vi "SetSRCreationDateStart(SubVI).vi"(10 "Date":timestamp, 11 "HTTP string":string) -> (3 "result string":string)   [LabVIEW 2018, in "Controller.lvlib"]
uses:
  Controller.lvlib
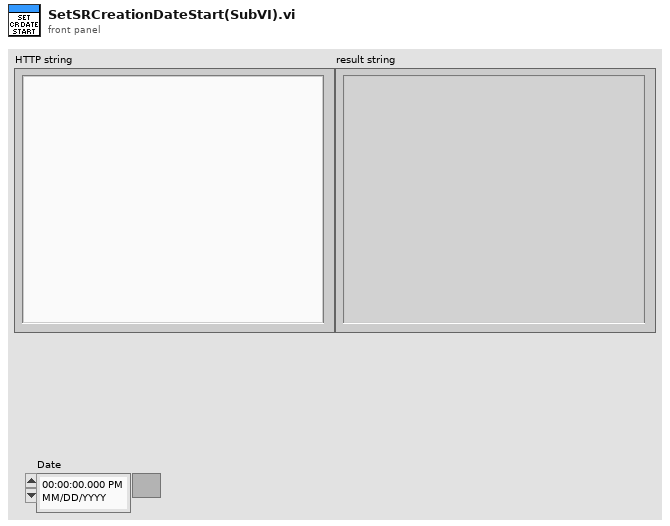
[diagram p1: front panel]
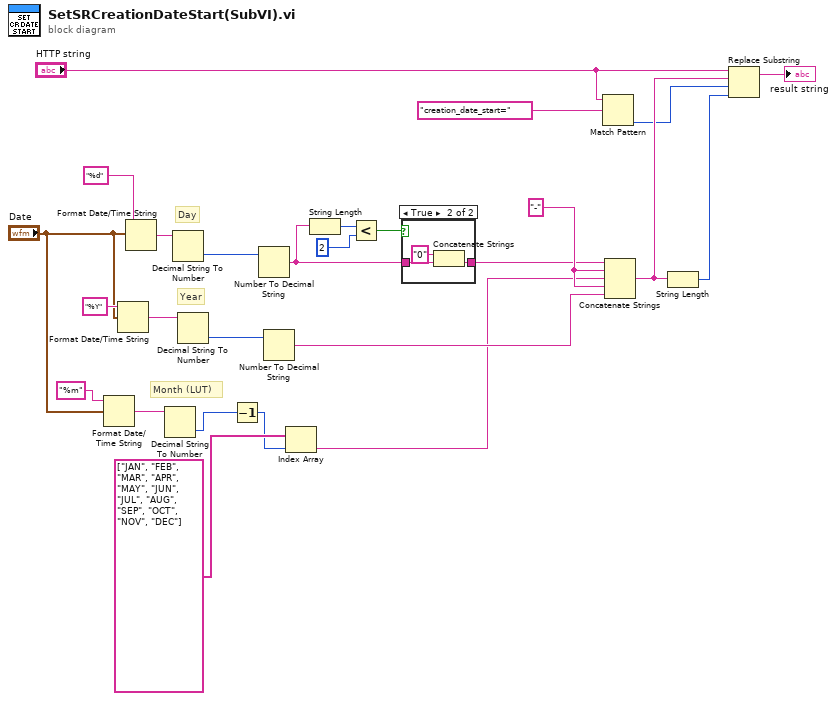
[diagram p0: block diagram]
diagram:
  w20 = "-" ("string")
  # "Month (LUT)"
  # "Year"
  # "Day"
  n1 = Format Date/Time String(time format string (%c)="%m", seconds (now)="Date") -> (date/time string=w6:string)  [unwired: 1 in]
  n2 = Format Date/Time String(time format string (%c)="%Y", seconds (now)="Date") -> (date/time string=w23:string)  [unwired: 1 in]
  n3 = Format Date/Time String(time format string (%c)="%d", seconds (now)="Date") -> (date/time string=w16:string)  [unwired: 1 in]
  n4 = Decimal String To Number(string=w6) -> (number=w2:i32)  [unwired: 2 in, 1 out]
  n5 = Decimal String To Number(string=w16) -> (number=w10:i32)  [unwired: 2 in, 1 out]
  n6 = Decimal String To Number(string=w23) -> (number=w9:i32)  [unwired: 2 in, 1 out]
  n7 = Decrement(x=w2) -> (x-1=w1:i32)
  n8 = Number To Decimal String(number=w10) -> (decimal integer string=w12:string)  [unwired: 1 in]
  n9 = Number To Decimal String(number=w9) -> (decimal integer string=w24:string)  [unwired: 1 in]
  n10 = Index Array(array=string[] ["JAN", "FEB", "MAR", "APR", "MAY", "JUN", "JUL", "AUG", "SEP", "OCT", "NOV", "DEC"], index=w1) -> (element=w4:string)
  n11 = String Length(string=w12) -> (length=w15:i32)
  n12 = Less?(x=w15, y=2) -> (x < y?=w13:bool)
  n13 = case shown="True" w13 {
    tunnel: w12 -> [w27 w30]
    tunnel: [w27 w28] -> w11
    frame False {
    }
    frame True {
      n14 = Concatenate Strings("0" ("string"), w30) -> (w28:string)
    }
  }
  n15 = Match Pattern(string="HTTP string", regular expression="creation_date_start=") -> (offset past match=w18:i32)  [unwired: 1 in, 3 out]
  n16 = Concatenate Strings(w11, w20, w4, w20, w24) -> (w25:string)
  n17 = String Length(string=w25) -> (length=w19:i32)
  n18 = Replace Substring(2:w19, 3:w18, 4:w25, 5:"HTTP string") -> (1:→"result string":string)  [unwired: 1 out]
